vi "readI16.vi"(8 "error in (no error)":errorcluster, 11 "II16Control in":refnum<class "II16Control.lvclass">) -> (0 "error out":errorcluster, 2 "Data":i16, 3 "II16Control out":refnum<class "II16Control.lvclass">)   [LabVIEW 2016, in "RTFPGA.lvlib" / "II16Control.lvclass"]
uses:
  II16Control.lvclass
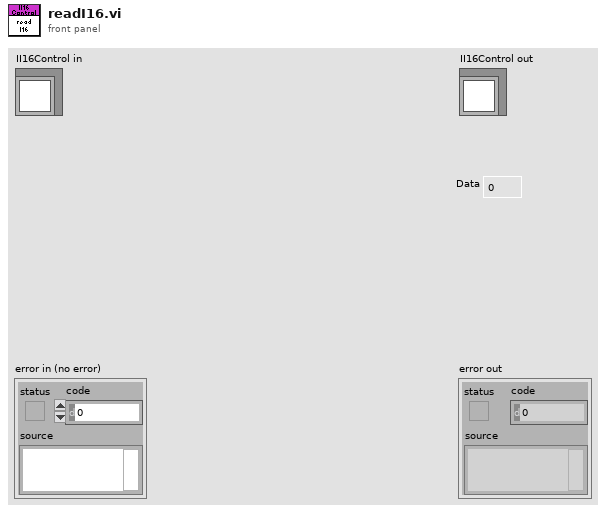
[diagram p1: front panel]
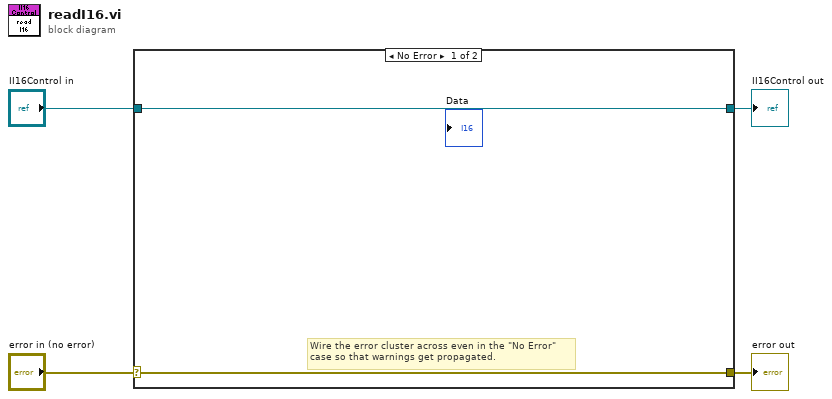
[diagram p0: block diagram]
diagram:
  n1 = case shown="No Error" "error in (no error)" {
    selector: "error in (no error)" -> [w5 w8]
    tunnel: [w5 w8] -> w3
    tunnel: [w6 w7] -> w1
    tunnel: "II16Control in" -> [w6 w7]
    frame No Error {
      # "Wire the error cluster across even in the \"No Error\"\ncase so that warnings get propagated."
    }
    frame Error {
    }
  }
  "error out" <- w3
  "II16Control out" <- w1
